vi "Load_Destination_Type.vi"(8 "error in (no error)":errorcluster, 9 "index":string, 11 "buildObject":T1) -> (0 "error out":errorcluster, 1 "index out":string, 3 "IB_Destination out":refnum<class "IB_Destination.lvclass">)   [LabVIEW 2020, in "IB_Destination.lvclass"]
uses:
  <vilib>/AppBuilder/IB_Classes/Destination/IB_Destination.lvclass
  <vilib>/AppBuilder/IB_Classes/Destination/IB_Destination.lvclass/IB_Destination.ctl
  <vilib>/AppBuilder/IB_Classes/Destination/absFolder/absFolder.lvclass
  <vilib>/AppBuilder/IB_Classes/Destination/userFolder/userFolder.lvclass
  <vilib>/AppBuilder/IB_Classes/Dest_User_NIPath/Dest_User_NIPath.lvclass
  <vilib>/AppBuilder/IB_Classes/Dest_User_MSIPath/Dest_User_MSIPath.lvclass
  e:/builds/penguin/labview/branches/2020/dev/dist/vi.lib/AppBuilder/IB_Classes/Destination/IB_Destination.lvclass
  e:/builds/penguin/labview/branches/2020/dev/dist/vi.lib/AppBuilder/IB_Classes/Destination/absFolder/absFolder.lvclass
  e:/builds/penguin/labview/branches/2020/dev/dist/vi.lib/AppBuilder/IB_Classes/Destination/userFolder/userFolder.lvclass
  e:/builds/penguin/labview/branches/2020/dev/dist/vi.lib/AppBuilder/IB_Classes/Destination/userLabel/userLabel.lvclass
  e:/builds/penguin/labview/branches/2020/dev/dist/vi.lib/AppBuilder/IB_Classes/Dest_User_NIPath/Dest_User_NIPath.lvclass
  e:/builds/penguin/labview/branches/2020/dev/dist/vi.lib/AppBuilder/IB_Classes/Dest_User_MSIPath/Dest_User_MSIPath.lvclass
  <resource>/Framework/Providers/API/ItemRef.ctl
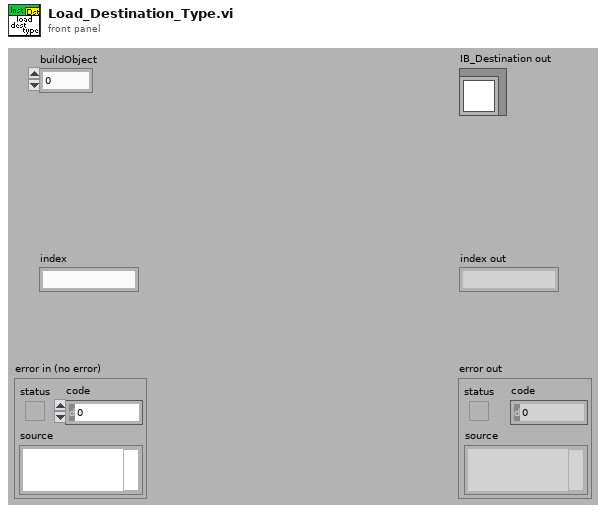
[diagram p1: front panel]
types:
  T1 = typedef "ItemRef.ctl" = u64
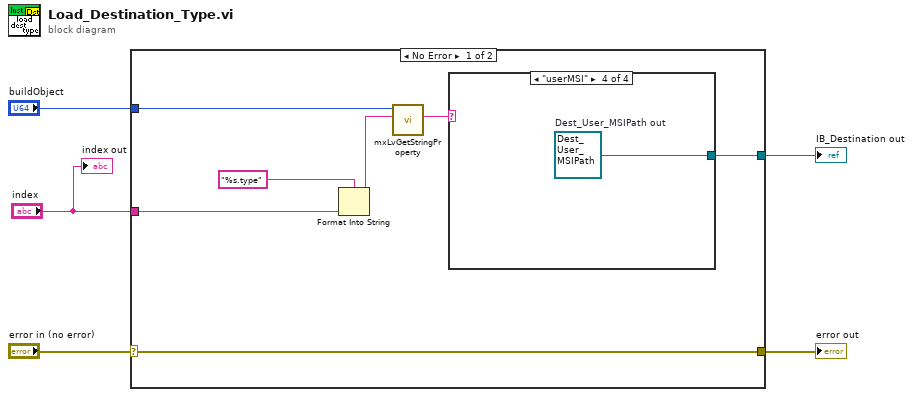
[diagram p0: block diagram]
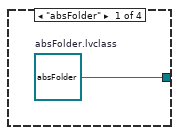
[diagram p2: hidden frame]
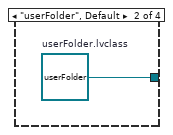
[diagram p3: hidden frame]
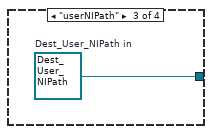
[diagram p4: hidden frame]
diagram:
  n1 = case shown="No Error" "error in (no error)" {
    selector: "error in (no error)" -> [w12 w17]
    tunnel: [w12 w17] -> w4
    tunnel: "buildObject" -> [w9 _]
    tunnel: "index" -> [w8 _]
    tunnel: [w6 _] -> w2
    frame No Error {
      n2 = Format Into String(format string="%s.type", w8) -> (resulting string=w11:string)  [unwired: 2 in, 1 out]
      n3 = call <resource>:"mxLvGetStringProperty.vi"("Tag"=w11, "Item"=w9) -> ("Value"=w7:string)  [unwired: 1 in, 8 out]
      n4 = case shown="\"userMSI\"" w7 {
        tunnel: [w13 w14 w15 w16] -> w6
        frame "absFolder" {
          w13 = refnum<class "absFolder.lvclass"> refnum  # absFolder.lvclass
        }
        frame "userFolder", Default {
          w14 = refnum<class "userFolder.lvclass"> refnum  # userFolder.lvclass
        }
        frame "userNIPath" {
          w15 = refnum<class "Dest_User_NIPath.lvclass"> refnum  # Dest_User_NIPath in
        }
        frame "userMSI" {
          w16 = refnum<class "Dest_User_MSIPath.lvclass"> refnum  # Dest_User_MSIPath out
        }
      }
    }
    frame Error {
    }
  }
  "error out" <- w4
  "IB_Destination out" <- w2
  "index out" <- "index"
